vi "main.vi"() -> ()   [LabVIEW 2016]
uses:
  <vilib>/Instr/_visa.llb/VISA Configure Serial Port (Instr).vi
panel:
  out "In Sync":bool
  out "L5":u32
  out "L4":u32
  out "L3":u32
  out "L2":u32
  out "L1":u32
  out "string length":dbl
  out "Random Number":i32(graph)
  out "status":bool
  out "error out":errorcluster
  in  "error in":errorcluster
  in  "instr name":string="Arduino"
  in  "write":bool
  in  "buffer size":u32=256
  in  "timeout (ms)":u32=10000
  in  "flow control":u16
  in  "stop bits":u16=10
  in  "parity":u16(ring) items=["None", "Odd", "Even", "Mark", "Space"]
  in  "data bits":u16=8 min=5 max=8 step=1
  in  "baud rate":u32=9600
  out "read string":string
  in  "write string":string
  in  "stop":bool
  # "Arduino LabVIEW - Serial Read and Write"
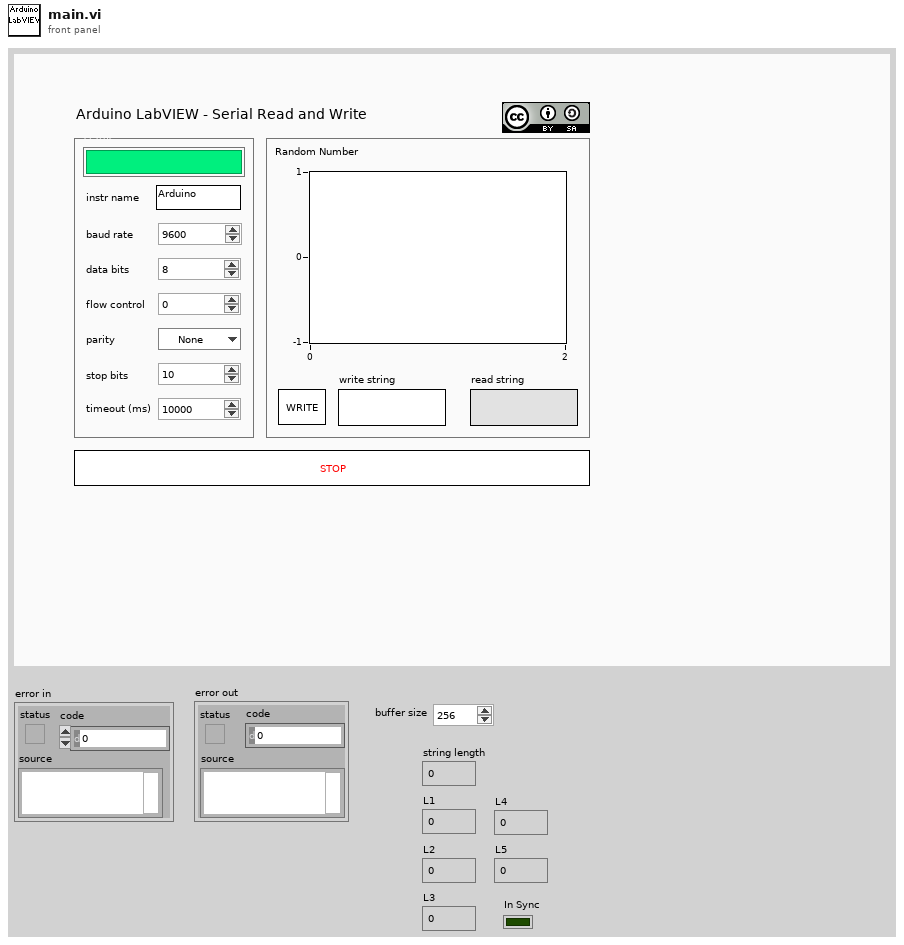
[diagram p1: front panel]
types:
  T1 = cluster{u16, u16, u16, u16, u16, u16, u16, u16, u16, u16}
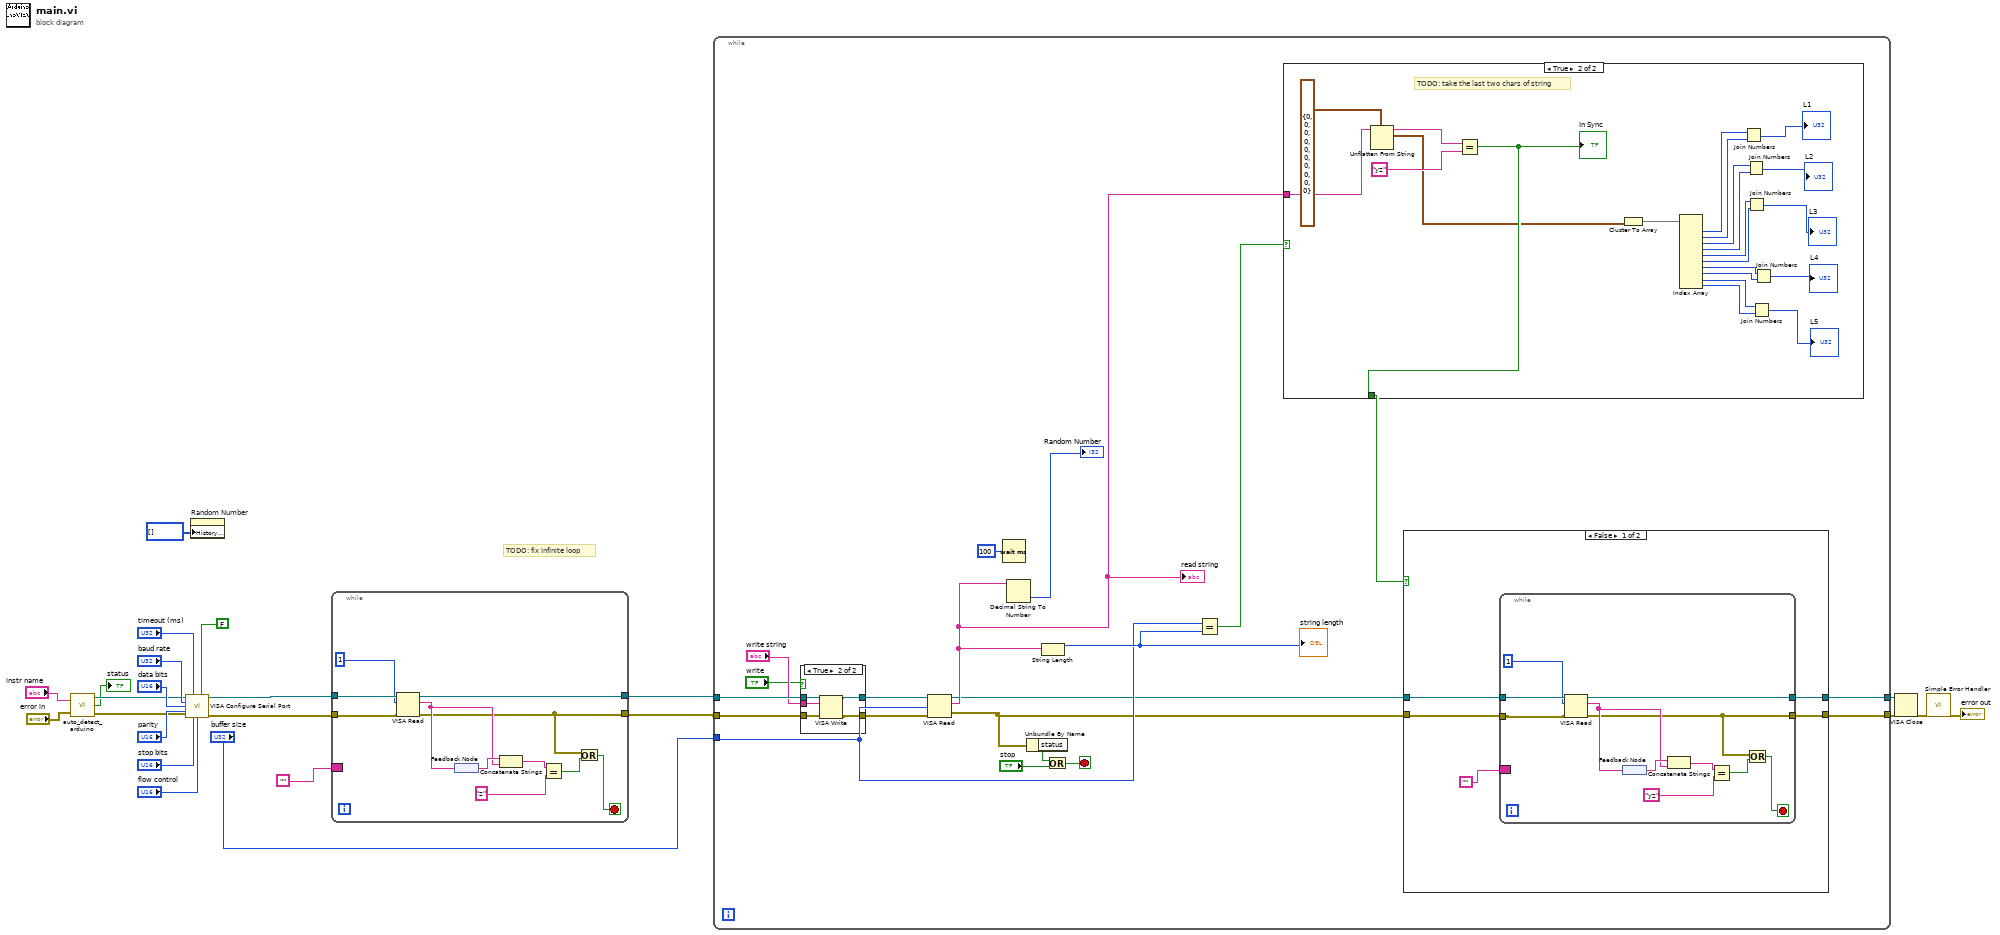
[diagram p0: block diagram]
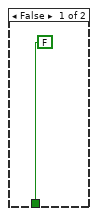
[diagram p3: hidden frame]
diagram:
  # "TODO: fix infinite loop"
  n1 = call "auto_detect_arduino.vi"("instr name"="instr name", "error in"="error in") -> ("VISA resource name"=w15:refnum<visa-resource-name>, "status"=→"status":bool, "error out"=w14:errorcluster)
  n2 = call-poly "VISA Configure Serial Port"("VISA resource name"=w15, "timeout (10sec)"="timeout (ms)", "Enable Termination\nChar (T)"=FALSE, "baud rate (9600)"="baud rate", "data bits (8)"="data bits", "parity (0:none)"="parity", "error in (no error)"=w14, "stop bits (10: 1 bit)"="stop bits", "flow control (0:none)"="flow control") -> ("VISA resource name out"=w6:refnum<visa-resource-name>, "error out"=w4:errorcluster)  [unwired: 5 in]
  n3 = property on="Random Number" class="WFChart (strict)"("History Data"=i32[] []) -> ()  [unwired: 2 in, 2 out]
  n4 = while {
    tunnel: w6 -> [w34]
    tunnel: [w33] -> w5
    tunnel: w4 -> [w32]
    tunnel: [w25] -> w3
    border: "" -> [_]
    stop <- w24 stop-if-true
    n5 = VISA Read(VISA resource name=w34, byte count=1, error in (no error)=w32) -> (VISA resource name out=w33:refnum<visa-resource-name>, read buffer=w29:string, error out=w25:errorcluster)  [unwired: 1 out]
    n6 = feedback-in #1(w29) -> ()
    n7 = feedback #1() -> (w30:string)
    n8 = Concatenate Strings(w30, w29) -> (w28:string)
    n9 = Equal?(x=w28, y="z") -> (x = y?=w26:bool)
    n10 = Or(x=w25, y=w26) -> (x .or. y?=w24:bool)
  }
  n11 = while {
    tunnel: w5 -> [w51]
    tunnel: w3 -> [w50]
    tunnel: [w39] -> w23
    tunnel: [w38] -> w22
    tunnel: "buffer size" -> [w42]
    stop <- w52 stop-if-true
    n12 = case shown="True" "write" {
      tunnel: w51 -> [w97 w102]
      tunnel: w50 -> [w96 w101]
      tunnel: [w97 w100] -> w49
      tunnel: [w96 w99] -> w48
      tunnel: "write string" -> [_ w98]
      frame False {
      }
      frame True {
        n13 = VISA Write(VISA resource name=w102, write buffer=w98, error in (no error)=w101) -> (VISA resource name out=w100:refnum<visa-resource-name>, error out=w99:errorcluster)  [unwired: 1 out]
      }
    }
    n14 = VISA Read(VISA resource name=w49, byte count=w42, error in (no error)=w48) -> (VISA resource name out=w36:refnum<visa-resource-name>, read buffer=w40:string, error out=w37:errorcluster)  [unwired: 1 out]
    "read string" <- w40
    n15 = Wait (ms)(milliseconds to wait=u32 100) -> ()  [unwired: 1 out]
    n16 = Decimal String To Number(string=w40) -> (number=→"Random Number":i32)  [unwired: 2 in, 1 out]
    n17 = Unbundle By Name(w37) -> ("status"=w54:bool)
    n18 = String Length(string=w40) -> (length=w43:i32)
    "string length" <- w43
    n19 = Or(x=w54, y="stop") -> (x .or. y?=w52:bool)
    n20 = Equal?(x=w42, y=w43) -> (x = y?=w41:bool)
    n21 = case shown="True" w41 {
      tunnel: w40 -> [_ w94]
      tunnel: [FALSE w91] -> w35
      frame False {
      }
      frame True {
        # "TODO: take the last two chars of string"
        n22 = Unflatten From String(type=T1 {0, 0, 0, 0, 0, 0, 0, 0, 0, 0}, binary string=w94) -> (rest of the binary string=w92:string, value=w90:T1)  [unwired: 3 in, 1 out]
        n23 = Equal?(x=w92, y="yz") -> (x = y?=w91:bool)
        "In Sync" <- w91
        n24 = Cluster To Array(cluster=w90) -> (array=w89:u16[])
        n25 = Index Array(array=w89) -> (element #1=w88:u16, element #2=w87:u16, element #3=w86:u16, element #4=w85:u16, element #5=w84:u16, element #6=w83:u16, element #7=w82:u16, element #8=w81:u16, element #9=w80:u16, element #10=w79:u16)  [unwired: 10 in]
        n26 = Join Numbers(hi=w88, lo=w87) -> ((hi.lo)=→"L1":u32)
        n27 = Join Numbers(hi=w86, lo=w85) -> ((hi.lo)=→"L2":u32)
        n28 = Join Numbers(hi=w84, lo=w83) -> ((hi.lo)=→"L3":u32)
        n29 = Join Numbers(hi=w80, lo=w79) -> ((hi.lo)=→"L5":u32)
        n30 = Join Numbers(hi=w82, lo=w81) -> ((hi.lo)=→"L4":u32)
      }
    }
    n31 = case shown="False" w35 {
      tunnel: [w58 w72] -> w39
      tunnel: [w57 w71] -> w38
      tunnel: w37 -> [w56 w71]
      tunnel: w36 -> [w55 w72]
      frame False {
        n32 = while {
          tunnel: w55 -> [w70]
          tunnel: [w69] -> w58
          tunnel: w56 -> [w68]
          tunnel: [w61] -> w57
          border: "" -> [_]
          stop <- w60 stop-if-true
          n33 = VISA Read(VISA resource name=w70, byte count=1, error in (no error)=w68) -> (VISA resource name out=w69:refnum<visa-resource-name>, read buffer=w65:string, error out=w61:errorcluster)  [unwired: 1 out]
          n34 = feedback-in #2(w65) -> ()
          n35 = feedback #2() -> (w66:string)
          n36 = Concatenate Strings(w66, w65) -> (w64:string)
          n37 = Equal?(x=w64, y="yz") -> (x = y?=w62:bool)
          n38 = Or(x=w61, y=w62) -> (x .or. y?=w60:bool)
        }
      }
      frame True {
      }
    }
  }
  n39 = VISA Close(VISA resource name=w23, error in (no error)=w22) -> (error out=w11:errorcluster)
  n40 = call <vilib>:"Simple Error Handler.vi"("error in (no error)"=w11) -> ("error out"=→"error out":errorcluster)  [unwired: 4 in, 4 out]
